vi "JJMCclase7.vi"() -> ()   [LabVIEW 2011]
panel:
  out "menor":dbl
  out "mayor":dbl
  out "promedio":dbl
  out "Thermometer":i32(slide) scale=0.0..100.0
  # "genrar 10 temperaturas y al finalpresentar la temperatura mayor, menor y la temperatura promedio"
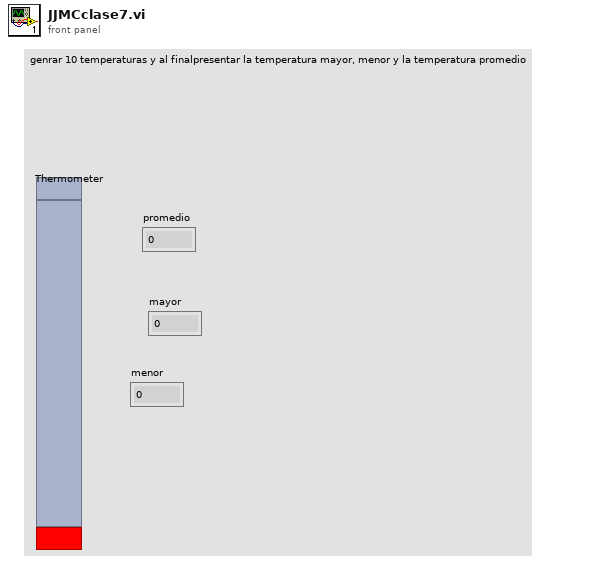
[diagram p1: front panel]
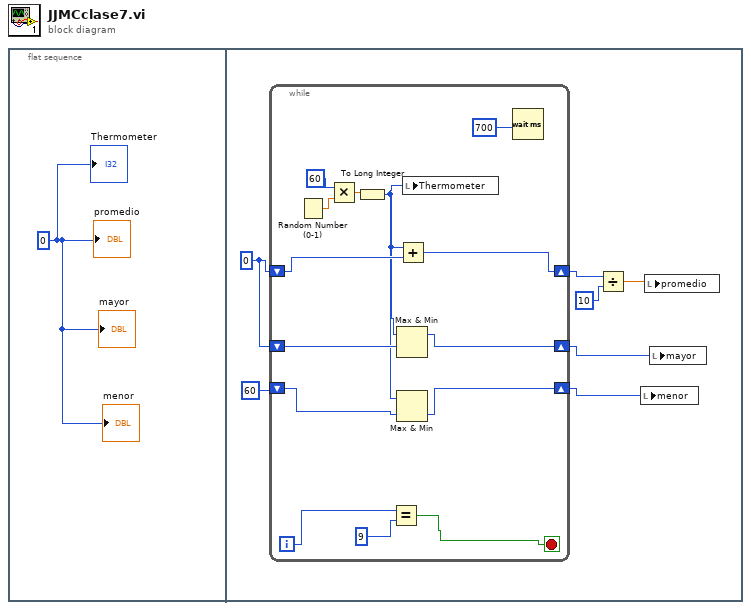
[diagram p0: block diagram]
diagram:
  n1 = flat-sequence {
    frame #0 {
      w1 = 0
      "Thermometer" <- w1
      "promedio" <- w1
      "mayor" <- w1
      "menor" <- w1
    }
    frame #1 {
      w4 = 0
      n2 = while {
        shift-right: [w16] -> w8
        shift-left: w4 -> [w15]
        shift-right: [w12] -> w5
        shift-left: w4 -> [w13]
        shift-right: [w9] -> w3
        shift-left: 60 -> [w11]
        i -> [w22]
        stop <- w20 stop-if-true
        n3 = Random Number (0-1)() -> (number: 0 to 1=w19:dbl)
        n4 = Multiply(x=60, y=w19) -> (x*y=w18:dbl)
        n5 = To Long Integer(number=w18) -> (32bit integer=w10:i32)
        n6 = Equal?(x=w22, y=9) -> (x = y?=w20:bool)
        n7 = Max & Min(x=w10, y=w13) -> (max(x,y)=w12:i32)  [unwired: 1 out]
        n8 = Max & Min(x=w10, y=w11) -> (min(x,y)=w9:i32)  [unwired: 1 out]
        n9 = Add(x=w10, y=w15) -> (x+y=w16:i32)
        n10 = local write "Thermometer"(w10) -> ()
        n11 = Wait (ms)(milliseconds to wait=700) -> ()  [unwired: 1 out]
      }
      n12 = Divide(x=w8, y=10) -> (x/y=w6:dbl)
      n13 = local write "menor"(w3) -> ()
      n14 = local write "promedio"(w6) -> ()
      n15 = local write "mayor"(w5) -> ()
    }
  }
